vi "event structure use.vi"() -> ()   [LabVIEW 2010]
panel:
  out "String 2":string
  in  "Boolean":bool
  out "String":string
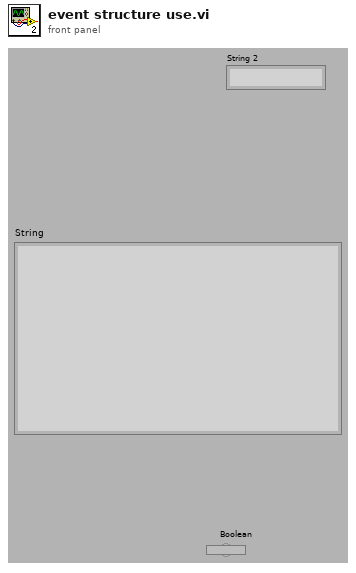
[diagram p1: front panel]
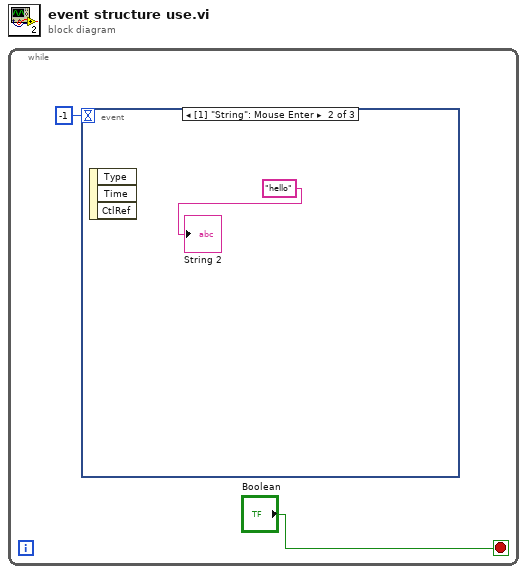
[diagram p0: block diagram]
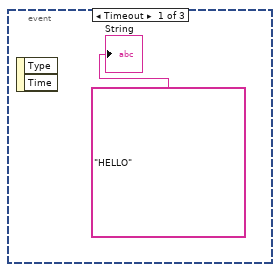
[diagram p2: hidden frame]
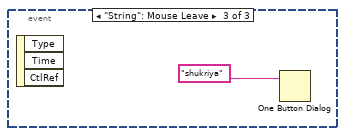
[diagram p3: hidden frame]
diagram:
  n1 = while {
    stop <- "Boolean" stop-if-true
    n2 = event shown="[1] \"String\": Mouse Enter" {
      selector: _ -> [_ _ _]
      dyn-events: _ -> [_ _ _]
      timeout: -1 -> [_ _ _]
      event Timeout {
        n3 = event-data() -> ()  [unwired: 1 in, 2 out]
        "String" <- "HELLO"
      }
      event "String": Mouse Enter {
        n4 = event-data() -> ()  [unwired: 1 in, 3 out]
        "String 2" <- "hello" ("String 2")
      }
      event "String": Mouse Leave {
        n5 = event-data() -> ()  [unwired: 1 in, 3 out]
        n6 = One Button Dialog(message="shukriya") -> ()  [unwired: 1 in, 1 out]
      }
    }
  }
